vi "RT-RIOtoVolt.vi"(1 "Rio-In":u16) -> (0 "Volt-Out":dbl)   [LabVIEW 2020]
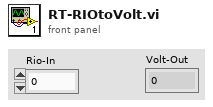
[diagram p1: front panel]
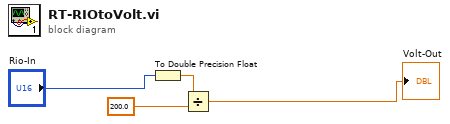
[diagram p0: block diagram]
diagram:
  n1 = To Double Precision Float(number="Rio-In") -> (double precision float=w2:dbl)
  n2 = Divide(x=w2, y=200.0) -> (x/y=→"Volt-Out":dbl)
